vi "FlattenCases.vi"(10 "Frame Names":string[](array[string])) -> (1 "diagram index":i32[](array[numeric]), 2 "cases":string[](array[string]))   [LabVIEW 2014, in "CaseStructure.lvclass"]
uses:
  CaseStructure.lvclass
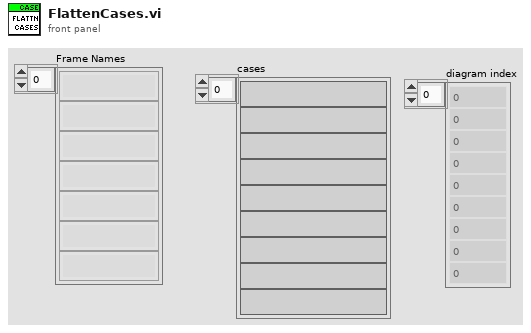
[diagram p1: front panel]
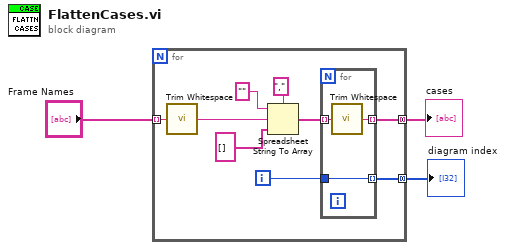
[diagram p0: block diagram]
diagram:
  n1 = for {
    tunnel: "Frame Names" -> [w12] mode=indexing
    tunnel: [w6] -> w2 mode=concatenating
    tunnel: [w5] -> w1 mode=concatenating
    i -> [w7]
    n2 = call <vilib>:"Trim Whitespace.vi"("string"=w12) -> ("trimmed string"=w4:string)  [unwired: 1 in]
    n3 = Spreadsheet String To Array(delimiter (Tab)=",", format string="", spreadsheet string=w4, array type (2D Dbl)=string[] []) -> (array=w8:string[])
    n4 = for {
      tunnel: w8 -> [w15] mode=indexing
      tunnel: w7 -> [w14]
      tunnel: [w13] -> w6 mode=indexing
      tunnel: [w14] -> w5 mode=indexing
      n5 = call <vilib>:"Trim Whitespace.vi"("string"=w15) -> ("trimmed string"=w13:string)  [unwired: 1 in]
    }
  }
  "cases" <- w2
  "diagram index" <- w1
